vi "Get_Test_Data_To_MES.vi"(1 "所有测试数据":string[][](array[string])=[["SN", "NA", "NA", "NA", "NA", "NA", "NA", "NA", "NA", ""], ["AC(mA)", "54", "42", "654", "354", "34", "543", "25", "45", ""], ["IR(Mohm)", "54", "42", "654", "354", "34", "543", "25", "45", ""], ["Result", "PASS", "FAIL", "PASS", "FAIL", "PASS", "FAIL", "FAIL", "FAIL", ""], ["", "", "", "", "", "", "", "", "", "NA"]]) -> (15 "数组":string[](array[string]), 16 "SN":string[](array[string]), 17 "RESULT":string[](array[string]))   [LabVIEW 2018]
panel:
  out "数组 2":string[][](array[string])
  out "所有测试数据 3":string[][](array[string])
  # "<Message>LowerLimit=5 UpperLimit=5.5 value=0</Message>"
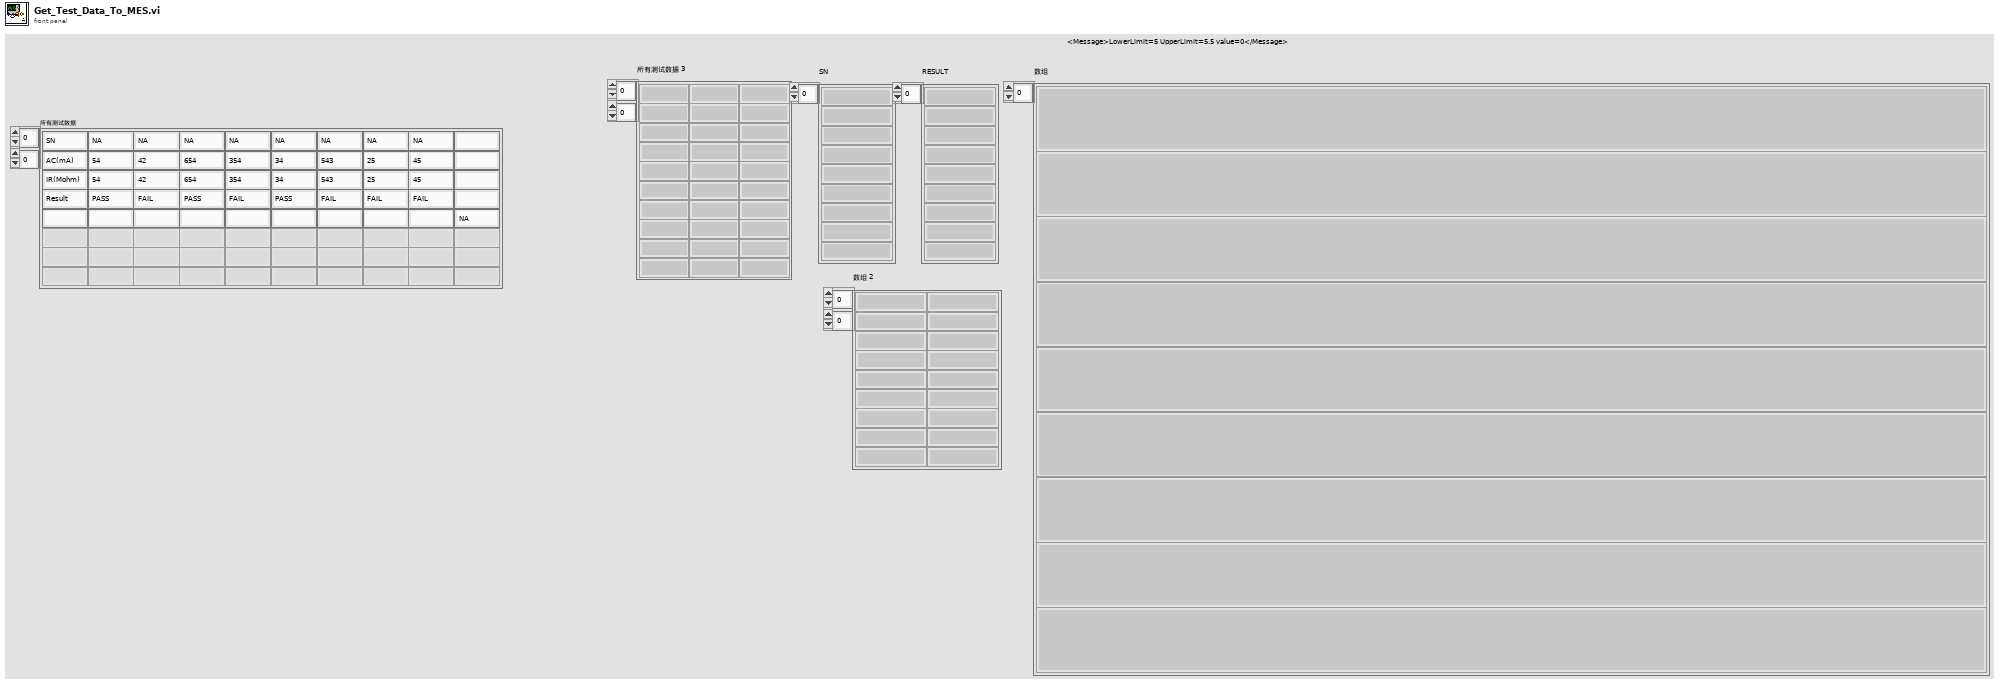
[diagram p1: front panel]
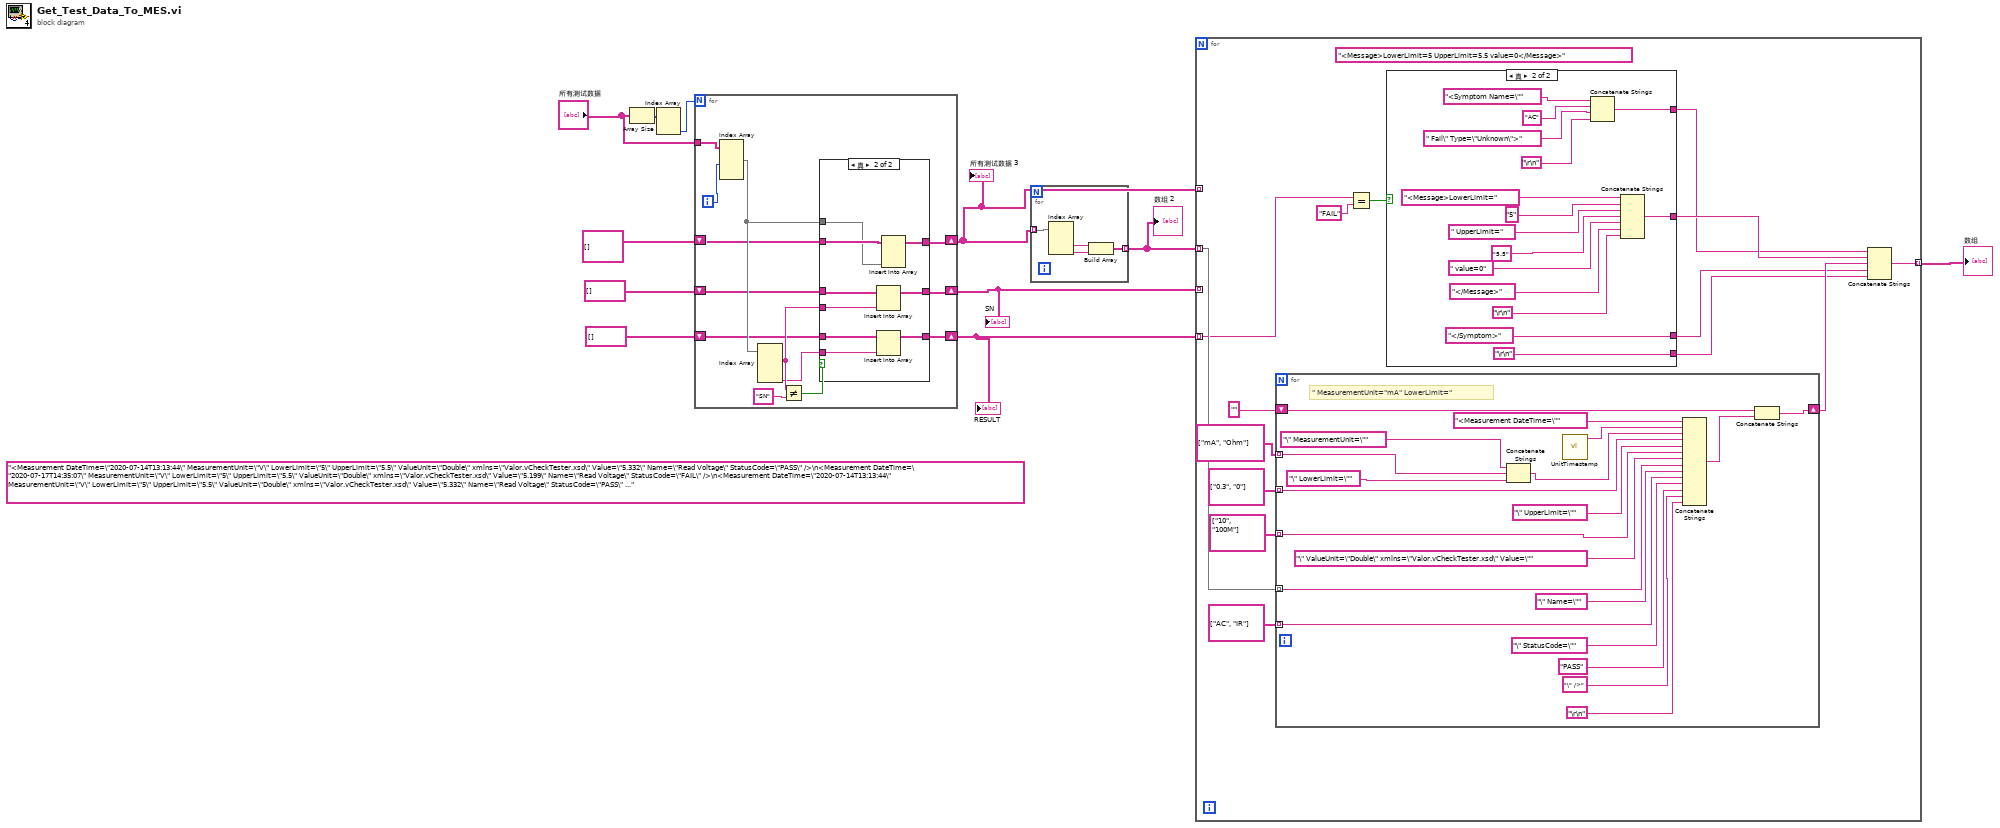
[diagram p0: block diagram]
diagram:
  (unwired) "<Measurement DateTime=\"2020-07-14T13:13:44\" MeasurementUnit=\"V\" LowerLimit=\"5\" UpperLimit=\"5.5\" ValueUnit=\"Double\" xmlns=\"Valor.vCheckTester.xsd\" Value=\"5.332\" Name=\"Read Voltage\" StatusCode=\"PASS\" />\n<Measurement DateTime=\"2020-07-17T14:35:07\" MeasurementUnit=\"V\" LowerLimit=\"5\" UpperLimit=\"5.5\" ValueUnit=\"Double\" xmlns=\"Valor.vCheckTester.xsd\" Value=\"5.199\" Name=\"Read Voltage\" StatusCode=\"FAIL\" />\n<Measurement DateTime=\"2020-07-14T13:13:44\" MeasurementUnit=\"V\" LowerLimit=\"5\" UpperLimit=\"5.5\" ValueUnit=\"Double\" xmlns=\"Valor.vCheckTester.xsd\" Value=\"5.332\" Name=\"Read Voltage\" StatusCode=\"PASS\" />"
  n1 = Array Size(array="所有测试数据") -> (size(s)=w11:i32[])
  n2 = Index Array(array=w11) -> (element #2=w10:i32)  [unwired: 2 in, 1 out]
  n3 = for {
    N: w10 -> [_]
    tunnel: "所有测试数据" -> [w24]
    shift-right: [w19] -> w2
    shift-left: string[][] [] -> [w20]
    shift-right: [w15] -> w6
    shift-left: string[] [] -> [w17]
    shift-right: [w14] -> w5
    shift-left: string[] [] -> [w13]
    i -> [w23]
    n4 = Index Array(array=w24, index (col) #1=w23) -> (element #1=w21:string[])  [unwired: 3 in, 1 out]
    n5 = Index Array(array=w21) -> (element #1=w16:string, element #4=w12:string)  [unwired: 4 in, 2 out]
    n6 = Not Equal?(x=w16, y="SN") -> (x != y?=w18:bool)
    n7 = case shown="真" w18 {
      tunnel: w21 -> [_ w34]
      tunnel: w20 -> [w27 w36]
      tunnel: [w27 w35] -> w19
      tunnel: w17 -> [w26 w33]
      tunnel: w16 -> [_ w32]
      tunnel: [w26 w31] -> w15
      tunnel: [w25 w30] -> w14
      tunnel: w13 -> [w25 w29]
      tunnel: w12 -> [_ w28]
      frame False {
      }
      frame True {
        n8 = Insert Into Array(array=w33, new element=w32) -> (w31:string[])  [unwired: 1 in]
        n9 = Insert Into Array(array=w29, new element=w28) -> (w30:string[])  [unwired: 1 in]
        n10 = Insert Into Array(array=w36, new element=w34) -> (w35:string[][])  [unwired: 2 in]
      }
    }
  }
  "所有测试数据 3" <- w2
  "SN" <- w6
  "RESULT" <- w5
  n11 = for {
    tunnel: w2 -> [w40] mode=indexing
    tunnel: [w37] -> w1 mode=indexing
    n12 = Index Array(array=w40) -> (element #2=w39:string, element #3=w38:string)  [unwired: 3 in, 1 out]
    n13 = Build Array(w39, w38) -> (w37:string[])
  }
  "数组 2" <- w1
  n14 = for {
    tunnel: w6 -> [_] mode=indexing
    tunnel: w5 -> [w42] mode=indexing
    tunnel: [w53] -> w3 mode=indexing
    tunnel: w2 -> [_] mode=indexing
    tunnel: w1 -> [w48] mode=indexing
    (unwired) "<Message>LowerLimit=5 UpperLimit=5.5 value=0</Message>"
    n15 = for {
      shift-right: [w80] -> w51
      shift-left: "" -> [w81]
      tunnel: string[] ["AC", "IR"] -> [w78] mode=indexing
      tunnel: w48 -> [w77] mode=indexing
      tunnel: string[] ["0.3", "0"] -> [w76] mode=indexing
      tunnel: string[] ["10", "100M"] -> [w75] mode=indexing
      tunnel: string[] ["mA", "Ohm"] -> [w73] mode=indexing
      # "\" MeasurementUnit=\"mA\" LowerLimit=\""
      n16 = Concatenate Strings("\" MeasurementUnit=\"", w73, "\" LowerLimit=\"") -> (w71:string)
      n17 = call "UnitTimestamp.vi"() -> ("字符串"=w89:string)  [unwired: 10 in, 1 out]
      n18 = Concatenate Strings("<Measurement DateTime=\"", w89, w71, w76, "\" UpperLimit=\"", w75, "\" ValueUnit=\"Double\" xmlns=\"Valor.vCheckTester.xsd\" Value=\"", w77, "\" Name=\"", w78, "\" StatusCode=\"", "PASS", "\" />", "\r\n") -> (w79:string)
      n19 = Concatenate Strings(w81, w79) -> (w80:string)
    }
    n20 = Equal?(x=w42, y="FAIL") -> (x = y?=w43:bool)
    n21 = case shown="真" w43 {
      tunnel: [_ w59] -> w55
      tunnel: [_ w58] -> w54
      tunnel: [_ "</Symptom>"] -> w50
      tunnel: [_ "\r\n"] -> w45
      frame False {
      }
      frame True {
        n22 = Concatenate Strings("<Symptom Name=\"", "AC", " Fail\" Type=\"Unknown\">", "\r\n") -> (w58:string)
        n23 = Concatenate Strings("<Message>LowerLimit=", "5", " UpperLimit=", "5.5", " value=0", "</Message>", "\r\n") -> (w59:string)
      }
    }
    n24 = Concatenate Strings(w54, w55, w51, w50, w45) -> (w53:string)
  }
  "数组" <- w3
